vi "Apply All Configurations.vi"(8 "error in (no error)":errorcluster, 11 "MotionSystem in":refnum<class "MotionSystem.lvclass">) -> (0 "error out":errorcluster, 3 "MotionSystem out":refnum<class "MotionSystem.lvclass">)   [LabVIEW 2016, in "MotionSystem.lvlib" / "MotionSystem.lvclass"]
uses:
  <userlib>/Common Components/Hardware/Abstract System/MotionSystem/MotionSystem/MotionSystem.lvclass
  <userlib>/Common Components/Hardware/Abstract System/MotionSystem/MotionSystem/MotionSystem.lvclass/MotionSystem.ctl
  <userlib>/Common Components/Hardware/Motor/Motor/Motor.lvclass
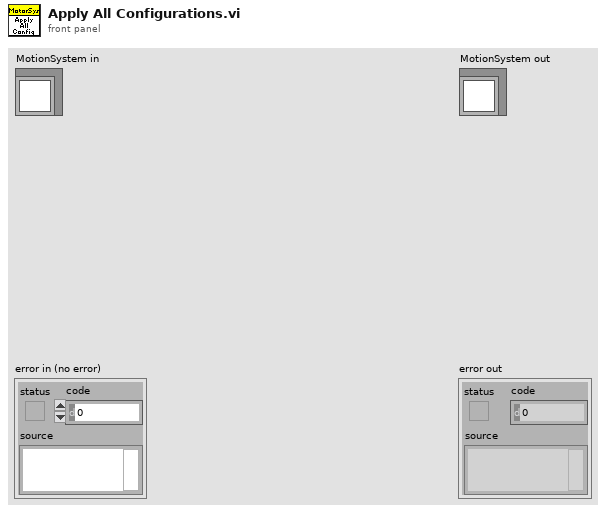
[diagram p1: front panel]
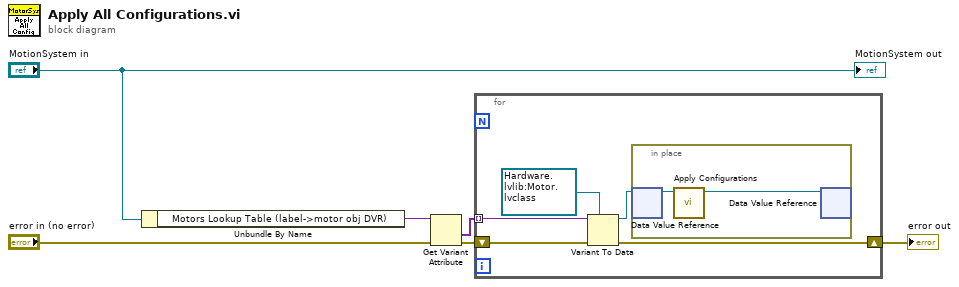
[diagram p0: block diagram]
diagram:
  n1 = Unbundle By Name("MotionSystem in") -> ("Motors Lookup Table (label->motor obj DVR)"=w6:variant)
  n2 = Get Variant Attribute(Variant=w6, error in="error in (no error)") -> (values=w5:variant[], error out=w4:errorcluster)  [unwired: 2 in, 2 out]
  n3 = for {
    tunnel: w5 -> [w11] mode=indexing
    shift-right: [w9] -> w2
    shift-left: w4 -> [w10]
    n4 = Variant To Data(error in=w10, type=refnum<data-value> refnum ("data value reference"), Variant=w11) -> (data=w7:refnum<data-value>, error out=w9:errorcluster)
    n5 = in-place {
      n6 = in-place-dvr #1(w7) -> (w13:refnum<class "Motor.lvclass">)  [unwired: 1 out]
      n7 = call-dynamic "Apply Configurations.vi"("Motor in"=w13) -> ("Motor out"=w12:refnum<class "Motor.lvclass">)  [unwired: 9 in, 1 out]
      n8 = in-place-dvr #1(w12) -> ()  [unwired: 2 out]
    }
  }
  "error out" <- w2
  "MotionSystem out" <- "MotionSystem in"
